vi "Plot Frequency Response - direct.vi"(0 "samples":i32=201, 1 "use dB":bool, 2 "b, forward coefficients":dbl[](array[numeric]), 3 "a, reverse coefficients":dbl[](array[numeric])=[1.0], 4 "unwrap":bool) -> (5 "Magnitude":cluster{dbl[], dbl[]}(graph), 6 "Phase":cluster{dbl[], dbl[]}(graph), 7 "Group Delay":cluster{dbl[], dbl[]}(graph))   [LabVIEW 2016]
doc: "Plot the frequency response of a filter described by its direct-form \"a\" (reverse) and \"b\" (forward) coefficients."
uses:
  <vilib>/Analysis/1siggen.llb/Ramp Pattern by Samples.vi
  <vilib>/Analysis/polynomials.llb/1D Polynomial Evaluation (CDB).vi
  <vilib>/Analysis/NI_AALBase.lvlib
  <vilib>/Analysis/NI_AALPro.lvlib
panel:
  # "freqz_cascade.vi"
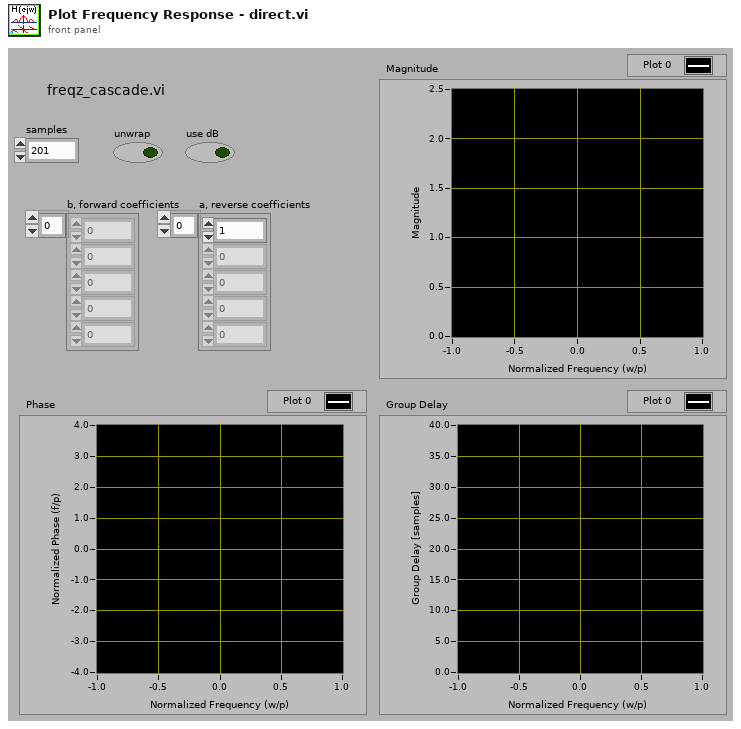
[diagram p1: front panel]
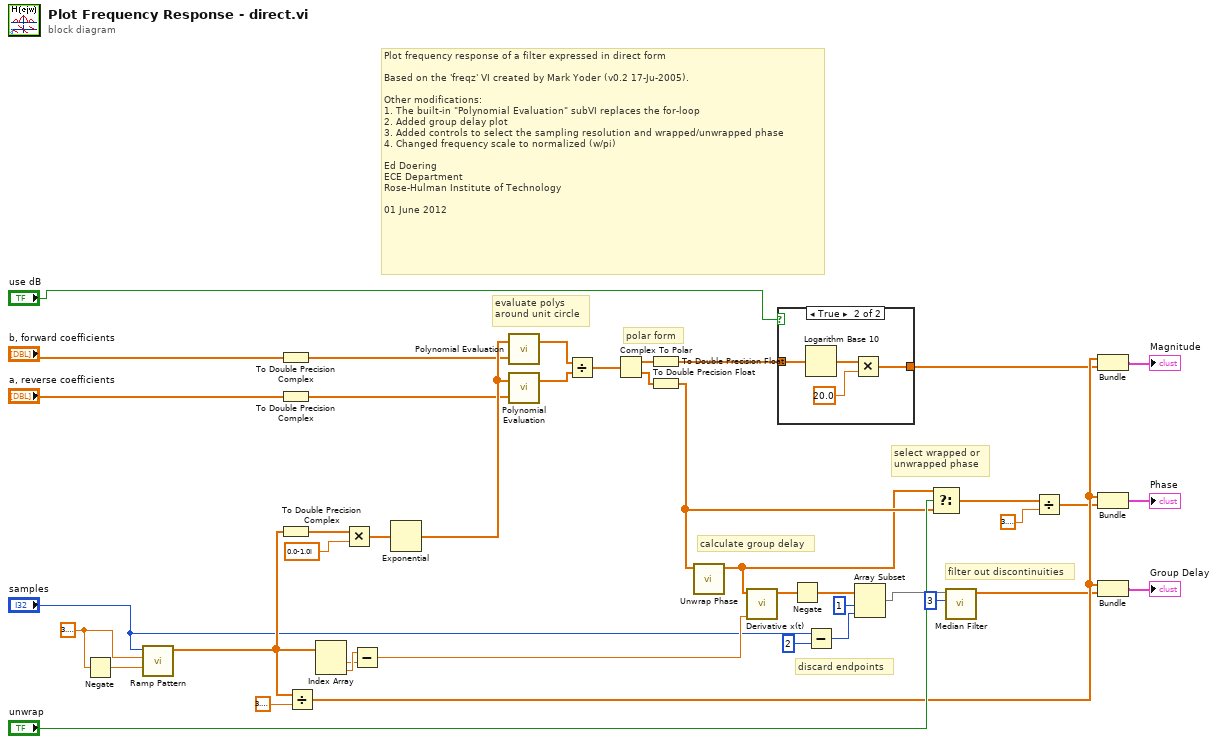
[diagram p0: block diagram]
diagram:
  w41 = 3.141592653589793
  # "filter out discontinuities"
  # "discard endpoints"
  # "evaluate polys\naround unit circle"
  # "polar form"
  # "select wrapped or\nunwrapped phase"
  # "calculate group delay"
  # "Plot frequency response of a filter expressed in direct form\n\nBased on the 'freqz' VI created by Mark Yoder (v0.2 17-Ju-2005).\n\nOther modifications:\n1. The built-in \"Polynomial Evaluation\" subVI replaces the for-loop\n2. Added group delay plot\n3. Added controls to select the sampling resolution and wrapped/unwrapped phase\n4. Changed frequency scale to normalized (w/pi)\n\nEd Doering\nECE Department\nRose-Hulman Institute of Technology\n\n01 June 2012"
  n1 = Negate(x=w41) -> (-x=w42:dbl)
  n2 = call-poly <vilib>:"Ramp Pattern.vi"("start"=w42, "end"=w41, "samples"="samples") -> ("Ramp Pattern"=w28:dbl[])  [unwired: 7 in, 1 out]
  n3 = To Double Precision Complex(1:"b, forward coefficients") -> (0:w13:cdb[])
  n4 = To Double Precision Complex(1:"a, reverse coefficients") -> (0:w12:cdb[])
  n5 = To Double Precision Complex(1:w28) -> (0:w36:cdb[])
  n6 = Divide(x=w28, y=3.141592653589793) -> (x/y=w23:dbl[])
  n7 = Index Array(array=w28) -> (element #1=w31:dbl, element #2=w32:dbl)  [unwired: 2 in]
  n8 = Multiply(x=w36, y=cdb 0.0-1.0i) -> (x*y=w38:cdb[])
  n9 = Subtract(x=w32, y=w31) -> (x-y=w30:dbl)
  n10 = Exponential(1:w38) -> (0:w35:cdb[])
  n11 = call-poly <vilib>:"Polynomial Evaluation.vi"("P(x)"=w13, "A"=w35) -> ("P(A)"=w16:cdb[])  [unwired: 1 out]
  n12 = call-poly <vilib>:"Polynomial Evaluation.vi"("P(x)"=w12, "A"=w35) -> ("P(A)"=w15:cdb[])  [unwired: 1 out]
  n13 = Divide(x=w16, y=w15) -> (x/y=w14:cdb[])
  n14 = Complex To Polar(r * e^(i*theta)=w14) -> (r=w40:dbl[], theta=w39:dbl[])
  n15 = To Double Precision Float(number=w40) -> (double precision float=w20:dbl[])
  n16 = To Double Precision Float(number=w39) -> (double precision float=w33:dbl[])
  n17 = call <vilib>:"Unwrap Phase.vi"("Phase"=w33) -> ("Unwrapped Phase"=w26:dbl[])  [unwired: 9 in, 1 out]
  n18 = call <vilib>:"Derivative x(t).vi"("dt"=w30, "X"=w26) -> ("dX/dt"=w29:dbl[])  [unwired: 8 in, 1 out]
  n19 = case shown="True" "use dB" {
    tunnel: w20 -> [w43 w45]
    tunnel: [w43 w44] -> w19
    frame False {
    }
    frame True {
      n20 = Logarithm Base 10(1:w45) -> (0:w46:dbl[])
      n21 = Multiply(x=w46, y=20.0) -> (x*y=w44:dbl[])
    }
  }
  n22 = Negate(x=w29) -> (-x=w10:dbl[])
  n23 = Subtract(x="samples", y=2) -> (x-y=w6:i32)
  n24 = Array Subset(array=w10, index=1, length=w6) -> (w9:dbl[])
  n25 = Select(t=w26, s="unwrap", f=w33) -> (s? t:f=w1:dbl[])
  n26 = call <vilib>:"Median Filter.vi"("left rank"=3, "X"=w9) -> ("Filtered X"=w11:dbl[])  [unwired: 8 in, 1 out]
  n27 = Divide(x=w1, y=3.141592653589793) -> (x/y=w3:dbl[])
  n28 = Bundle(w23, w19) -> (→"Magnitude":cluster{dbl[], dbl[]})  [unwired: 1 in]
  n29 = Bundle(w23, w3) -> (→"Phase":cluster{dbl[], dbl[]})  [unwired: 1 in]
  n30 = Bundle(w23, "Filtered X"=w11) -> (→"Group Delay":cluster{dbl[], "Filtered X":dbl[]})  [unwired: 1 in]
